vi "stop_approach_conditions.vi"(5 "z":dbl, 6 "max movement":dbl=5.0, 7 "Original z":dbl, 8 "SD Factor":dbl, 9 "Original SD":dbl, 10 "Original Mean":dbl, 11 "QPD Mean":dbl) -> (0 "Stop Condition":bool)   [LabVIEW 2019]
panel:
  in  "max desired piezo position":dbl=20.0
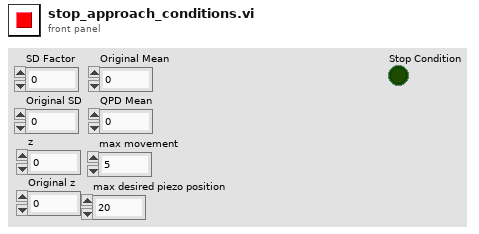
[diagram p1: front panel]
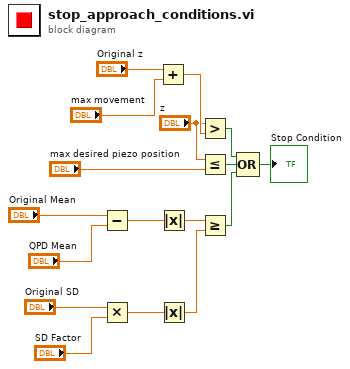
[diagram p0: block diagram]
diagram:
  n1 = Subtract(x="Original Mean", y="QPD Mean") -> (x-y=w17:dbl)
  n2 = Multiply(x="Original SD", y="SD Factor") -> (x*y=w5:dbl)
  n3 = Add(x="Original z", y="max movement") -> (x+y=w2:dbl)
  n4 = Absolute Value(x=w17) -> (abs(x)=w16:dbl)
  n5 = Absolute Value(x=w5) -> (abs(x)=w4:dbl)
  n6 = Greater?(x="z", y=w2) -> (0:w10:bool)
  n7 = Less Or Equal?(x="z", y="max desired piezo position") -> (x <= y?=w11:bool)
  n8 = Greater Or Equal?(x=w16, y=w4) -> (x >= y?=w9:bool)
  n9 = Compound Arithmetic op=OR(w10, w11, w9) -> (→"Stop Condition":bool)
